vi "Read datatype.vi"(8 "error in (no error)":errorcluster, 11 "JSON Object in":refnum<class "JSON Object.lvclass">) -> (0 "error out":errorcluster, 2 "datatype":T1, 3 "JSON Object out":refnum<class "JSON Object.lvclass">)   [LabVIEW 2016, in "LVJSON.lvlib" / "JSON Object.lvclass"]
doc: "Returns the JSON Type of the given object. This may be used to determine if the value of a control of type JSON Null, JSON Literal or JSON Structured Type is an instance of a more specific type."
uses:
  JSON Object.lvclass
  JSON Types.ctl
  LVJSON.lvlib
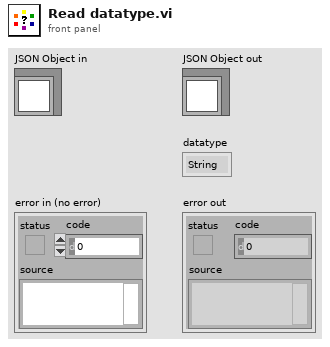
[diagram p1: front panel]
types:
  T1 = typedef "LVJSON.lvlib/JSON Types.ctl" = enum16{"String", "Numeric", "Boolean", "NULL", "Object", "Array"}
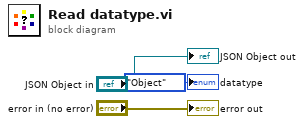
[diagram p0: block diagram]
diagram:
  "error out" <- "error in (no error)"
  "JSON Object out" <- "JSON Object in"
  "datatype" <- JSON_Types."Object" ("datatype")
